vi "Get Available Software 1.0.vi"   [LabVIEW 2017, in "nisyscfg.lvlib"]
doc: "Retrieves a list of software available on the local system."
uses:
  <vilib>/nisyscfg/nisyscfg.lvlib
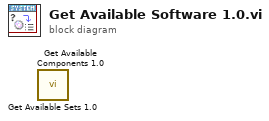
[diagram p0: block diagram]
diagram:
  n1 = call <vilib>:"Get Available Sets 1.0.vi"() -> ()  [unwired: 9 in, 3 out]
  n2 = call <vilib>:"Get Available Components 1.0.vi"() -> ()  [unwired: 9 in, 3 out]
